vi "HIL_Boost_PVP-HT.vi"(9 "u":bool, 11 "Entradas Boost_PVP":T2={"Irradiancia"=500.0, "¿conectado?"=FALSE}) -> (2 "Estados Boost_pvp_Vd":T1 {"x_1=V_D/a (V)" format="%^#_10g"})   [LabVIEW 2019]
uses:
  Ctl_VI/boost_PVP/Entradas boost.ctl
  Estados Boost_pvp_Vd.ctl
  <vilib>/rvi/FXPMathLib/FxpMul/XNode/nifxpmath_Multiplier.xnode
  <vilib>/rvi/FXPMathLib/FxpSub/XNode/nifxpmath_Sub.xnode
  <vilib>/rvi/FXPMathLib/FxpAdd/XNode/nifxpmath_Add.xnode
  <vilib>/rvi/FXPMathLib/sim/FxpSim.dll
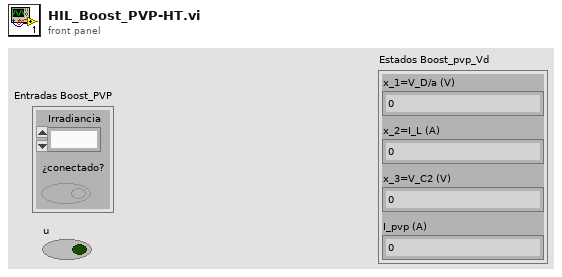
[diagram p1: front panel]
types:
  T1 = typedef "Estados Boost_pvp_Vd.ctl" = cluster{"x_1=V_D/a (V)":fxp<+,32,9>, "x_2=I_L (A)":fxp<+,32,6>, "x_3=V_C2 (V)":fxp<+,32,9>, "I_pvp (A)":fxp<+,32,4>}
  T2 = typedef "Entradas boost.ctl" = cluster{"Irradiancia":fxp<+,10,10>, "¿conectado?":bool}
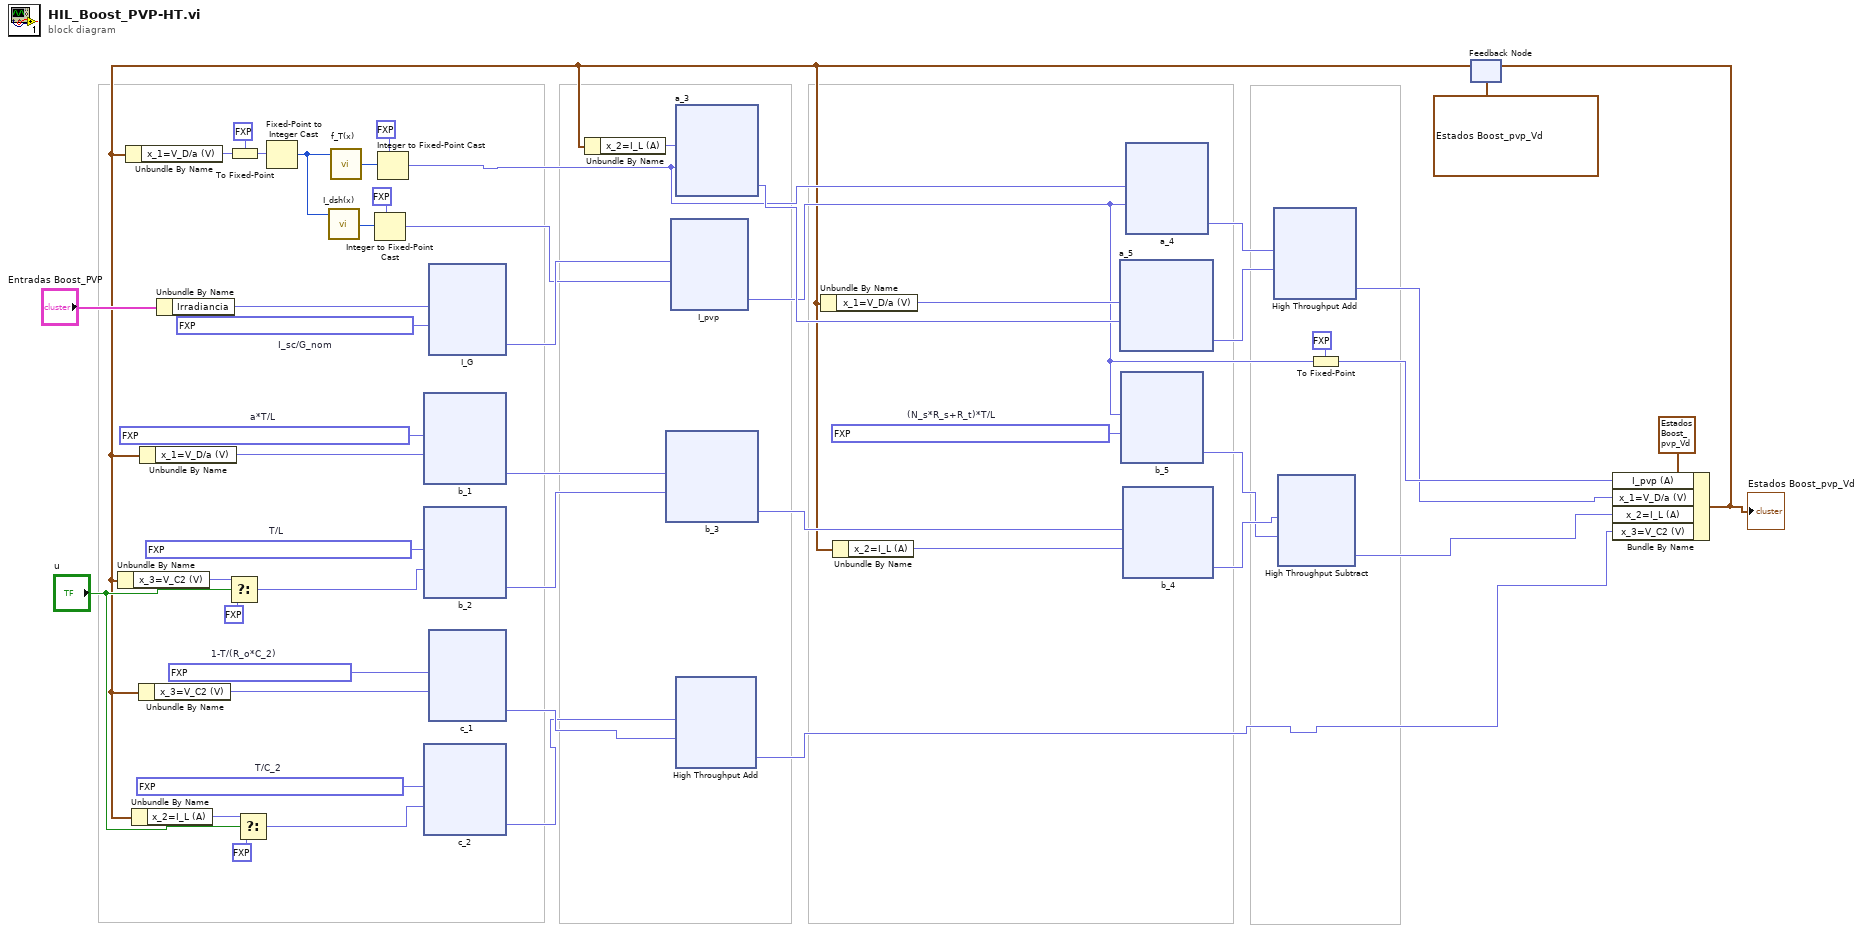
[diagram p0: block diagram]
diagram:
  w21 = fxp<+,32,-15> 1.6211317657166546e-05  # (N_s*R_s+R_t)*T/L
  w32 = fxp<+,32,-10> 0.000833333333275732  # T/C_2
  w33 = fxp<+,32,0> 0.9999977238476276  # 1-T/(R_o*C_2)
  w42 = fxp<+,32,-16> 7.812500001591616e-06  # T/L
  w43 = fxp<+,32,-17> 4.005676620622012e-06  # a*T/L
  w45 = fxp<+,32,-6> 0.00904004000040004  # I_sc/G_nom
  n1 = Unbundle By Name("Entradas Boost_PVP") -> ("Irradiancia"=w46:fxp<+,10,10>)
  n2 = xnode "I_G"("x"=w46, "y"=w45) -> ("x*y"=w26:fxp<+,42,4>)
  n3 = feedback #1(T1 {"x_1=V_D/a (V)"=18.292400002479553, "x_2=I_L (A)"=0.0, "x_3=V_C2 (V)"=0.0, "I_pvp (A)"=0.0} ("Estados Boost_pvp_Vd")) -> (w8:T1)
  n4 = Unbundle By Name(w8) -> ("x_3=V_C2 (V)"=w41:fxp<+,32,9>)
  n5 = Unbundle By Name(w8) -> ("x_1=V_D/a (V)"=w51:fxp<+,32,9>)
  n6 = Unbundle By Name(w8) -> ("x_2=I_L (A)"=w31:fxp<+,32,6>)
  n7 = Unbundle By Name(w8) -> ("x_3=V_C2 (V)"=w34:fxp<+,32,9>)
  n8 = Unbundle By Name(w8) -> ("x_1=V_D/a (V)"=w44:fxp<+,32,9>)
  n9 = Select(t=w41, s="u", f=fxp<+,32,9> 0.0) -> (s? t:f=w39:fxp<+,32,9>)
  n10 = To Fixed-Point(fixed-point type=fxp<+,14,9> 0.0, number=w51) -> (fixed-point=w49:fxp<+,14,9>)
  n11 = Select(t=w31, s="u", f=fxp<+,32,6> 0.0) -> (s? t:f=w30:fxp<+,32,6>)
  n12 = Fixed-Point to Integer Cast(1:w49) -> (0:w48:u16)
  n13 = call "I_dsh(x)"("address"=w48) -> ("data out"=w37:u32)  [unwired: 8 in]
  n14 = call "f_T(x)"("address"=w48) -> ("data out"=w38:u32)  [unwired: 8 in]
  n15 = Integer to Fixed-Point Cast(fixed-point type=fxp<+,32,4> 0.0, integer=w37) -> (fixed-point=w14:fxp<+,32,4>)
  n16 = Integer to Fixed-Point Cast(fixed-point type=fxp<+,32,-8> 0.0, integer=w38) -> (fixed-point=w13:fxp<+,32,-8>)
  n17 = xnode "b_1"("x"=w43, "y"=w44) -> ("x*y"=w25:fxp<+,64,-8>)
  n18 = xnode "b_2"("x"=w42, "y"=w39) -> ("x*y"=w24:fxp<+,64,-7>)
  n19 = xnode "c_2"("x"=w32, "y"=w30) -> ("x*y"=w9:fxp<+,64,-4>)
  n20 = xnode "c_1"("x"=w33, "y"=w34) -> ("x*y"=w10:fxp<+,64,9>)
  n21 = Unbundle By Name(w8) -> ("x_2=I_L (A)"=w27:fxp<+,32,6>)
  n22 = xnode "b_3"("x"=w25, "y"=w24) -> ("x-y"=w20:fxp<+/-,64,-5>)
  n23 = xnode "I_pvp"("x"=w26, "y"=w14) -> ("x-y"=w16:fxp<+,44,6>)
  n24 = xnode "a_3"("x"=w27, "y"=w13) -> ("x*y"=w23:fxp<+,64,-2>)
  n25 = xnode "High Throughput Add"("x"=w9, "y"=w10) -> ("x+y"=w3:fxp<+,32,9>)
  n26 = Unbundle By Name(w8) -> ("x_1=V_D/a (V)"=w22:fxp<+,32,9>)
  n27 = Unbundle By Name(w8) -> ("x_2=I_L (A)"=w19:fxp<+,32,6>)
  n28 = xnode "a_5"("x"=w22, "y"=w23) -> ("x-y"=w17:fxp<+/-,64,11>)
  n29 = xnode "b_5"("x"=w16, "y"=w21) -> ("x*y"=w6:fxp<+,64,-9>)
  n30 = xnode "b_4"("x"=w20, "y"=w19) -> ("x+y"=w7:fxp<+/-,64,8>)
  n31 = xnode "a_4"("x"=w13, "y"=w16) -> ("x*y"=w18:fxp<+,64,-2>)
  n32 = xnode "High Throughput Add"("x"=w18, "y"=w17) -> ("x+y"=w5:fxp<+,32,9>)
  n33 = xnode "High Throughput Subtract"("x"=w7, "y"=w6) -> ("x-y"=w4:fxp<+,32,6>)
  n34 = To Fixed-Point(fixed-point type=fxp<+,32,4> 0.0, number=w16) -> (fixed-point=w11:fxp<+,32,4>)
  n35 = Bundle By Name(cluster=T1 {"x_1=V_D/a (V)"=0.0, "x_2=I_L (A)"=0.0, "x_3=V_C2 (V)"=0.0, "I_pvp (A)"=0.0} ("Estados Boost_pvp_Vd"), "I_pvp (A)"=w11, "x_1=V_D/a (V)"=w5, "x_2=I_L (A)"=w4, "x_3=V_C2 (V)"=w3) -> (w2:T1)
  "Estados Boost_pvp_Vd" <- w2
  n36 = feedback-in #1(w2) -> ()
